vi "RunMeas.vi"(8 "error in (no error)":errorcluster, 11 "NHRDCPower in":refnum<class "NHRDCPower.lvclass">) -> (0 "error out":errorcluster, 2 "variant":variant, 3 "NHRDCPower out":refnum<class "NHRDCPower.lvclass">)   [LabVIEW 2018, in "AcPwrPlugins.lvlib" / "NHRDCPower.lvclass"]
doc: "This VI initiates and takes measurements from the instrument(s)."
uses:
  NHRDCPower.lvclass
  C:/Users/ico/Documents/Projects/NistPluggableModules/AcPwr/AcPwrPlugins/AcPwrBaseClass/AcPwrBase.lvclass
  <instrlib>/NHRDCPowerModule/NHRDCPowerModule/NHRDCPowerModule.lvlib
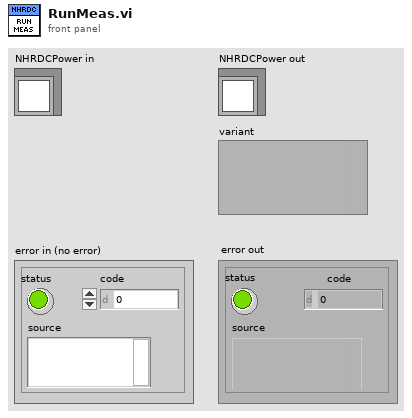
[diagram p1: front panel]
types:
  T1 = typedef "AcPwrPlugins.lvlib/NHRDCPower.lvclass/Measurements.ctl" = cluster{"Handle":string, "Name":string, "Enabled":bool, "Measurement Value":sgl, "btnMeasFetch":bool, "Measurement Type":i32, "Fetch Method":i32, "Fetch Time (s)":sgl}[]
  T2 = cluster{"Handle":string, "Name":string, "Enabled":bool, "Measurement Value":sgl, "btnMeasFetch":bool, "Measurement Type":i32, "Fetch Method":i32, "Fetch Time (s)":sgl}
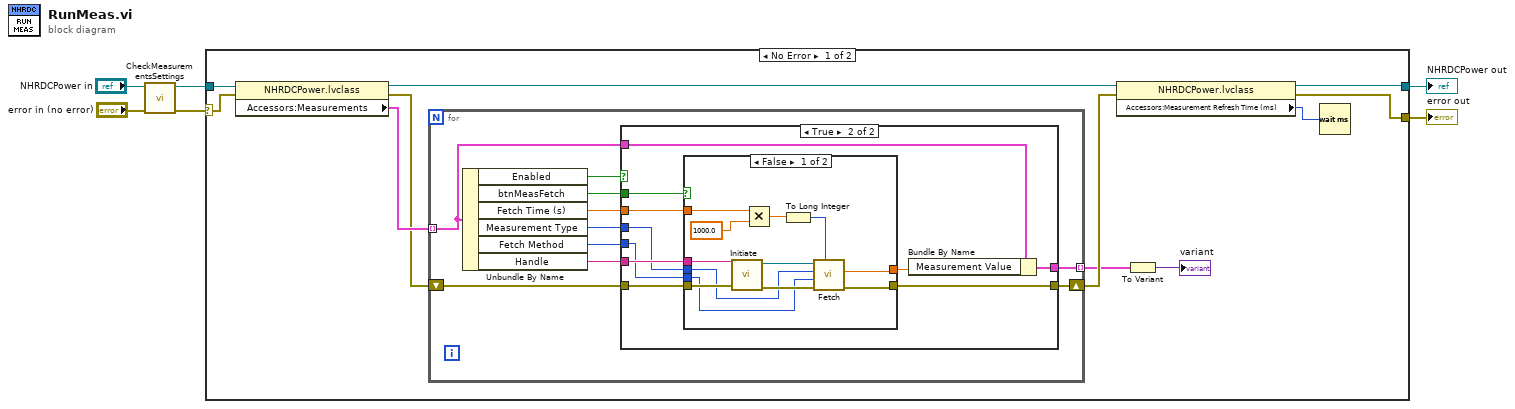
[diagram p0: block diagram]
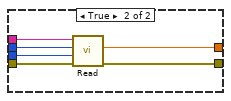
[diagram p3: hidden frame]
diagram:
  n1 = call-dynamic "CheckMeasurementsSettings.vi"("error in (no error)"="error in (no error)", "NHRDCPower in"="NHRDCPower in") -> ("error out"=w2:errorcluster, "NHRDCPower out"=w1:refnum<class "NHRDCPower.lvclass">)  [unwired: 8 in]
  n2 = case shown="No Error" w2 {
    selector: w2 -> [w16 w57]
    tunnel: [w10 w57] -> w6
    tunnel: [w11 w58] -> w5
    tunnel: w1 -> [w17 w58]
    frame No Error {
      n3 = property class="NHRDCPower.lvclass"(reference=w17, error in=w16) -> (reference out=w13:refnum<class "NHRDCPower.lvclass">, error out=w14:errorcluster, "Accessors:Measurements"=w15:T1)
      n4 = for {
        tunnel: w15 -> [w27] mode=indexing
        shift-right: [w24] -> w12
        shift-left: w14 -> [w26]
        tunnel: [w22] -> w8 mode=indexing
        n5 = Unbundle By Name(w27) -> ("Enabled"=w20:bool, "btnMeasFetch"=w23:bool, "Fetch Time (s)"=w18:sgl, "Measurement Type"=w21:i32, "Fetch Method"=w25:i32, "Handle"=w19:string)
        n6 = case shown="True" w20 {
          tunnel: w27 -> [_ w37]
          tunnel: w26 -> [w28 w36]
          tunnel: w25 -> [_ w32]
          tunnel: [w28 w35] -> w24
          tunnel: [_ w38] -> w22
          tunnel: w21 -> [_ w31]
          tunnel: w23 -> [_ w30]
          tunnel: w19 -> [_ w33]
          tunnel: w18 -> [_ w29]
          frame False {
          }
          frame True {
            n7 = case shown="False" w30 {
              tunnel: w36 -> [w50 w56]
              tunnel: [w45 w55] -> w35
              tunnel: [w46 w54] -> w34
              tunnel: w33 -> [w49 w53]
              tunnel: w32 -> [w44 w52]
              tunnel: w31 -> [w43 w51]
              tunnel: w29 -> [w41 _]
              frame False {
                n8 = call <instrlib>:"Initiate.vi"("error in (no error)"=w50, "instrument handle"=w49) -> ("error out"=w48:errorcluster, "instrument handle out"=w47:refnum<visa-resource-name>)  [unwired: 8 in]
                n9 = Multiply(x=w41, y=1000.0) -> (x*y=w40:dbl)
                n10 = To Long Integer(number=w40) -> (32bit integer=w39:i32)
                n11 = call <instrlib>:"Fetch.vi"("(infinite)"=w39, "error in (no error)"=w48, "method (Aperture)"=w44, "measurement (Voltage)"=w43, "instrument handle"=w47) -> ("error out"=w45:errorcluster, "measured value"=w46:sgl)  [unwired: 4 in, 1 out]
              }
              frame True {
                n12 = call <instrlib>:"Read.vi"("error in (no error)"=w56, "method (Aperture)"=w52, "measurement (Voltage)"=w51, "instrument handle"=w53) -> ("error out"=w55:errorcluster, "measured value"=w54:sgl)  [unwired: 5 in, 1 out]
              }
            }
            n13 = Bundle By Name(cluster=w37, "Measurement Value"=w34) -> (w38:T2)
          }
        }
      }
      n14 = property class="NHRDCPower.lvclass"(reference=w13, error in=w12) -> (reference out=w11:refnum<class "NHRDCPower.lvclass">, error out=w10:errorcluster, "Accessors:Measurement Refresh Time (ms)"=w9:u32)
      n15 = To Variant(anything=w8) -> (Variant=→"variant":variant)
      n16 = Wait (ms)(milliseconds to wait=w9) -> ()  [unwired: 1 out]
    }
    frame Error {
    }
  }
  "NHRDCPower out" <- w5
  "error out" <- w6
